vi "VI to Verify.vi"   [LabVIEW 2020]
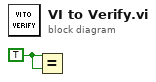
[diagram p0: block diagram]
diagram:
  w1 = TRUE
  n1 = Equal?(x=w1, y=w1) -> ()  [unwired: 1 out]
